vi "Do.vi"(8 "error in (no error)":errorcluster, 10 "Actor in":refnum<class "Actor.lvclass">, 11 "Send Get Hardware Info Message":refnum<class "Send Get Hardware Info Message.lvclass">) -> (0 "error out":errorcluster, 2 "Actor out":refnum<class "Actor.lvclass">)   [LabVIEW 2016, in "Controller UI.lvlib" / "Send Get Hardware Info Message.lvclass"]
uses:
  <userlib>/Common Components/Controller UI/Messages/Send Get Hardware Info Message/Send Get Hardware Info Message.lvclass
  <vilib>/ActorFramework/Actor/Actor.lvclass
  <userlib>/Common Components/Controller UI/Controller UI.lvclass
  C:/Program Files (x86)/National Instruments/LabVIEW 2016/vi.lib/ActorFramework/Actor/Actor.lvclass
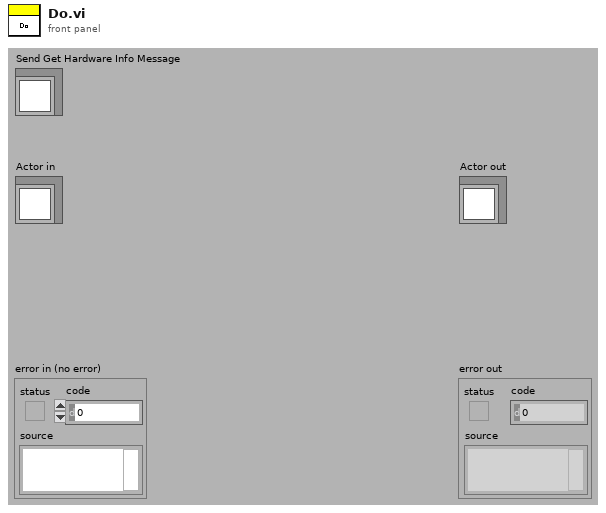
[diagram p1: front panel]
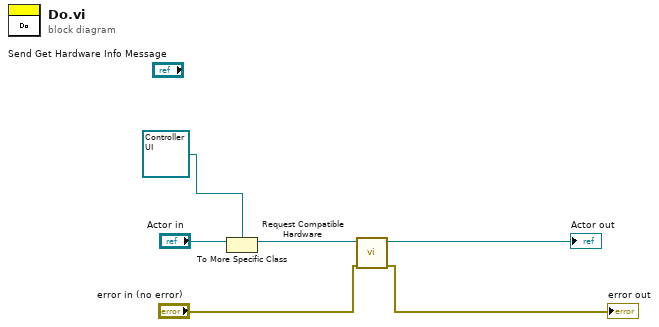
[diagram p0: block diagram]
diagram:
  n1 = To More Specific Class(target class=refnum<class "Controller UI.lvclass"> refnum ("UI.lvclass"), reference="Actor in") -> (specific class reference=w4:refnum<class "Controller UI.lvclass">)  [unwired: 1 in, 1 out]
  n2 = call-dynamic "Request Compatible Hardware.vi"("error in (no error)"="error in (no error)", "Fcn UI in"=w4) -> ("error out"=→"error out":errorcluster, "Fcn UI out"=→"Actor out":refnum<class "Controller UI.lvclass">)  [unwired: 8 in]
